vi "MouseMove_test.vi"() -> ()   [LabVIEW 2010]
uses:
  C:/Users/rshang/Desktop/MouseMove/MouseMove_LVandCsharp/ClassLibrary1.dll
  MouseMove/MouseMove_LVandCsharp/ClassLibrary1.dll
  <vilib>/Utility/error.llb/DialogType.ctl
panel:
  in  "ty":string="692"
  in  "tx":string="1247"
  in  "stop":bool
  out "GetMousePosition":string="816@364"
  in  "Boolean":bool=TRUE
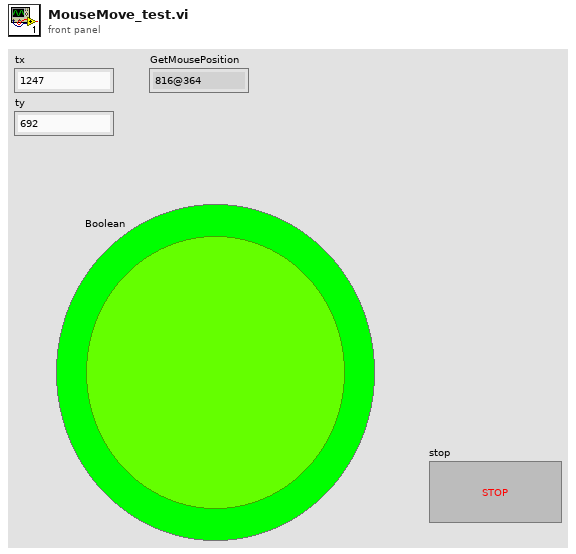
[diagram p1: front panel]
types:
  T1 = typedef "DialogType.ctl" = u16
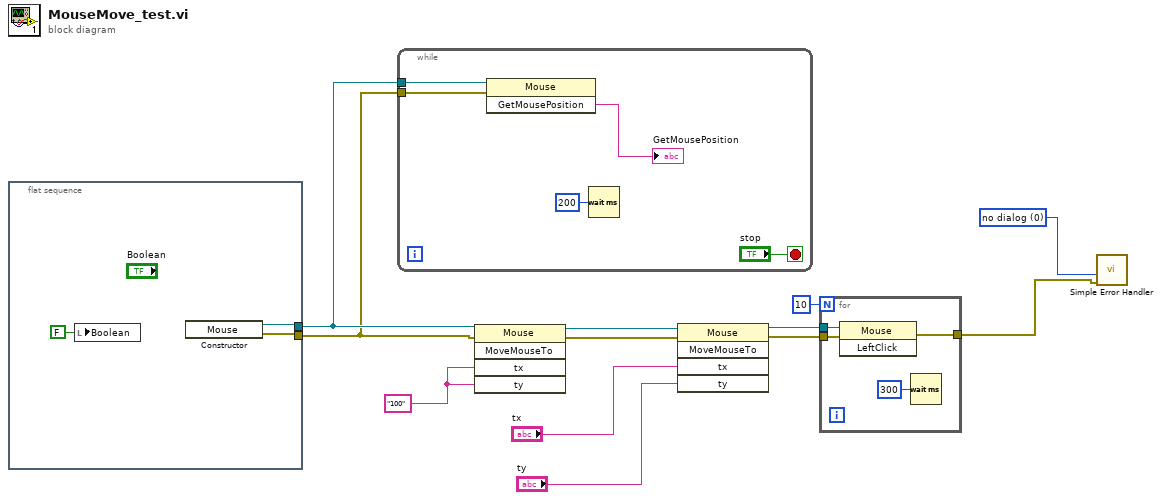
[diagram p0: block diagram]
diagram:
  w1 = T1 0 items=["no dialog", "OK message", "continue or stop message", "OK message + warnings", "continue/stop + warnings"] ("type of dialog (OK msg:1)")
  w12 = "100" ("tx")
  n1 = flat-sequence {
    tunnel: [w14] -> w11
    tunnel: [w13] -> w10
    frame #0 {
      n2 = local write "Boolean"(FALSE ("Boolean")) -> ()
      n3 = constructor class="Mouse"() -> (reference out=w14:refnum<k24>, error out=w13:errorcluster)  [unwired: 3 in, 1 out]
    }
  }
  n4 = while {
    tunnel: w11 -> [w20]
    tunnel: w10 -> [w19]
    stop <- "stop" stop-if-true
    n5 = invoke class="Mouse" method="GetMousePosition"(reference=w20, error in=w19) -> ("GetMousePosition"=→"GetMousePosition":string)  [unwired: 1 in, 2 out]
    n6 = Wait (ms)(milliseconds to wait=u32 200) -> ()  [unwired: 1 out]
  }
  n7 = invoke class="Mouse" method="MoveMouseTo"(reference=w11, error in=w10, "tx"=w12, "ty"=w12) -> (reference out=w9:refnum<k24>, error out=w8:errorcluster)  [unwired: 1 in, 3 out]
  n8 = invoke class="Mouse" method="MoveMouseTo"(reference=w9, error in=w8, "tx"="tx", "ty"="ty") -> (reference out=w5:refnum<k24>, error out=w4:errorcluster)  [unwired: 1 in, 3 out]
  n9 = for {
    N: 10 -> [_]
    tunnel: w5 -> [w24]
    tunnel: w4 -> [w23]
    tunnel: [w22] -> w2
    n10 = invoke class="Mouse" method="LeftClick"(reference=w24, error in=w23) -> (error out=w22:errorcluster)  [unwired: 1 in, 2 out]
    n11 = Wait (ms)(milliseconds to wait=u32 300) -> ()  [unwired: 1 out]
  }
  n12 = call <vilib>:"Simple Error Handler.vi"("type of dialog (OK msg:1)"=w1, "error in (no error)"=w2) -> ()  [unwired: 3 in, 5 out]
